vi "Operate Limit Switches.vi"(6 "True state":bool, 7 "Limit switch selector":enum16{"Limit switch 1", "Limit Switch 2"}(ring)=enum."Limit Switch 2", 8 "error in (no error)":errorcluster, 9 "Use switch?":bool, 10 "Index":i32, 11 "Visa Array in":refnum<visa-resource-name>[](array[refnum])) -> (0 "error out":errorcluster, 3 "Visa Array out":refnum<visa-resource-name>[](array[refnum]))   [LabVIEW 2010, in "SignalWriterMH110203USBStepperMotor.lvclass"]
uses:
  SignalWriterMH110203USBStepperMotor.lvclass
  class_data.vi
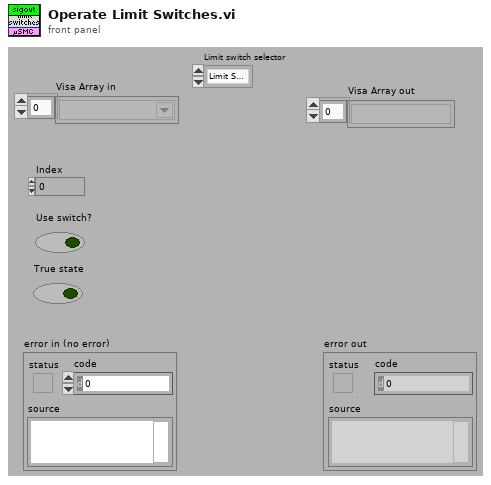
[diagram p1: front panel]
types:
  T1 = typedef "SignalWriterMH110203USBStepperMotor.lvclass/Mode Control (uSMC).ctl" = cluster{"Turn Buttons Off":bool, "Reduce Current":bool, "Power Off and Make a Whole Step":bool, "Emergency Power Off":bool, "Limit Switch 1 True State":bool, "Limit Switch 2 True State":bool, "Rotary Transducer TRUE State":bool, "Swap Limit Switches":bool, "Limit Switch 1 Operation Enabled":bool, "Limit Switch 2 Operation Enabled":bool, "Rotary Transducer Operation Enabled":bool, "Rotary Transducer Operation Select":bool, "Button 1 True State":bool, "Button 2 True State":bool, "Swap Buttons":bool, "Reset Rotary Transducer Check Positions":bool, "Output Syncronization Enabled":bool, "Reset Output Sync Count":bool, "Sync Operation":bool, "Sync Count":u32, "Power":bool, "Invert Sync Polarity":bool, "Use Encoder":bool, "Invert Encoder Direction":bool, "Reset Encoder To 0":bool, "Reset SM Enc Pos to Enc Pos":bool}
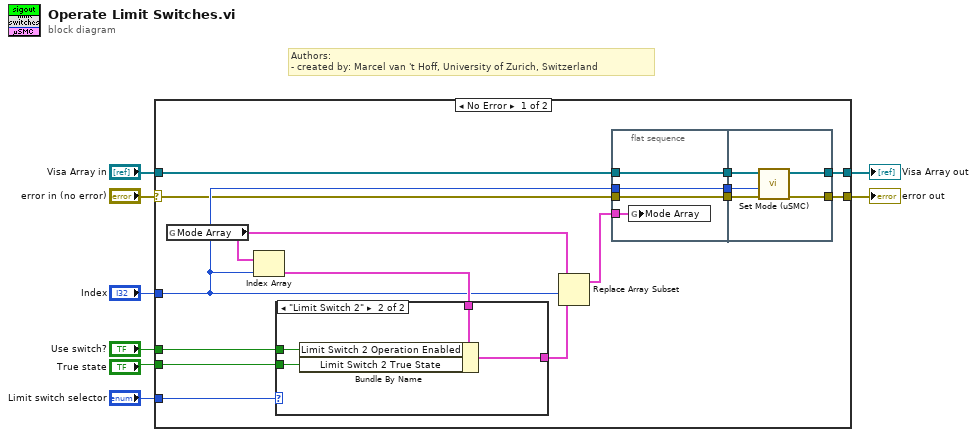
[diagram p0: block diagram]
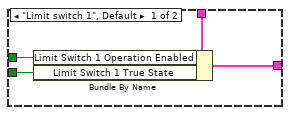
[diagram p2: hidden frame]
diagram:
  # "Authors: \n- created by: Marcel van 't Hoff, University of Zurich, Switzerland"
  n1 = case shown="No Error" "error in (no error)" {
    selector: "error in (no error)" -> [w9 w41]
    tunnel: "Visa Array in" -> [w20 w42]
    tunnel: [w19 w42] -> w7
    tunnel: [w18 w41] -> w6
    tunnel: "Use switch?" -> [w16 _]
    tunnel: "True state" -> [w15 _]
    tunnel: "Limit switch selector" -> [w14 _]
    tunnel: "Index" -> [w11 _]
    frame No Error {
      n2 = global read "class_data.vi" "Mode Array"() -> (w12:T1[])
      n3 = Index Array(array=w12, index=w11) -> (element=w17:T1)
      n4 = case shown="\"Limit Switch 2\"" w14 {
        tunnel: w17 -> [w36 w40]
        tunnel: w16 -> [w35 w38]
        tunnel: w15 -> [w34 w37]
        tunnel: [w33 w39] -> w13
        frame "Limit switch 1", Default {
          n5 = Bundle By Name(cluster=w36, "Limit Switch 1 Operation Enabled"=w35, "Limit Switch 1 True State"=w34) -> (w33:T1)
        }
        frame "Limit Switch 2" {
          n6 = Bundle By Name(cluster=w40, "Limit Switch 2 Operation Enabled"=w38, "Limit Switch 2 True State"=w37) -> (w39:T1)
        }
      }
      n7 = Replace Array Subset(array=w12, new element=w13, index=w11) -> (w10:T1[])
      n8 = flat-sequence {
        tunnel: w11 -> [w25]
        tunnel: w9 -> [w26]
        tunnel: w20 -> [w27]
        tunnel: [w27] -> w23
        tunnel: [w26] -> w22
        tunnel: [w25] -> w21
        tunnel: w10 -> [w24]
        tunnel: [w31] -> w19
        tunnel: [w29] -> w18
        tunnel: w23 -> [w32]
        tunnel: w22 -> [w30]
        tunnel: w21 -> [w28]
        frame #0 {
          n9 = global write "class_data.vi" "Mode Array"(w24) -> ()
        }
        frame #1 {
          n10 = call "Set Mode (uSMC).vi"("error in (no error)"=w30, "Index"=w28, "Visa Array in"=w32) -> ("error out"=w29:errorcluster, "Visa Array out"=w31:refnum<visa-resource-name>[])  [unwired: 7 in]
        }
      }
    }
    frame Error {
    }
  }
  "Visa Array out" <- w7
  "error out" <- w6
